vi "2.vi"() -> ()   [LabVIEW 2019]
uses:
  <vilib>/imath/engines/lvmath/Plug In/_Char/NIMS_CH_character datatype.ctl
  <vilib>/imath/engines/lvmath2/RunTimeEngine/RangeToken/NIMS_Range.vi
  <instcachedir>/0/NIMS_Range_FADF6ADDA3E145BB934C8BD4C7DAAB97.lvgen/NIMS_Range_FADF6ADDA3E145BB934C8BD4C7DAAB97_000.vi
  <vilib>/imathl/engines/lvmath/Functions/Error Handling/Create Error.vi
  <vilib>/imath/engines/lvmath/Plug In/_Char/NIMS_CH_Character RV to String.vi
  <vilib>/imath/engines/lvmath2/RunTimeEngine/BuiltInFunctions/random/NIMS_random.vi
  <vilib>/imath/engines/lvmath2/RunTimeEngine/IndexRead/NIMS M(S).vi
  <instcachedir>/0/NIMS M(S)_B826C018497E4940AE96BD27B540B6FB.lvgen/NIMS M(S)_B826C018497E4940AE96BD27B540B6FB_000.vi
  <vilib>/imath/engines/lvmath2/RunTimeEngine/ArithmeticOperatorToken/NIMS_ArithmeticOperator_plus.vi
  <instcachedir>/0/NIMS_ArithmeticOperator_plus_5C9385B0197D46E2B844C41E02F9EC39.lvgen/NIMS_ArithmeticOperator_plus_5C9385B0197D46E2B844C41E02F9EC39_004.vi
  <vilib>/imath/engines/lvmath2/RunTimeEngine/ErrorHandling/NIMS_Create Error From Enums.vi
  <vilib>/imath/engines/lvmath2/RunTimeEngine/BuiltInFunctions/randnormal/NIMS_randnormal(1,I32).vi
  <vilib>/imath/engines/lvmath2/RunTimeEngine/ErrorHandling/NIMS_Error From Error Code.vi
  <vilib>/imath/engines/lvmath/Functions/Error Handling/MergeErrorsWrapper.vi
  <vilib>/imath/engines/lvmath2/RunTimeEngine/BuiltInFunctions/crosscorr/NIMS_crosscorr(GM,Str).vi
  <instcachedir>/0/NIMS_crosscorr(GM,Str)_7E3A3CE9917B451394D0C3CD4C3D6955.lvgen/NIMS_crosscorr(GM,Str)_7E3A3CE9917B451394D0C3CD4C3D6955_000.vi
  <vilib>/imath/engines/lvmath2/RunTimeEngine/BuiltInFunctions/fft/NIMS_fft(GM).vi
  <instcachedir>/0/NIMS_fft(GM)_17D9014FFEBE444196AC5CE36A7D9342.lvgen/NIMS_fft(GM)_17D9014FFEBE444196AC5CE36A7D9342_000.vi
  <vilib>/imath/engines/lvmath2/RunTimeEngine/BuiltInFunctions/abs/NIMS_abs(signed).vi
  <instcachedir>/0/NIMS_abs(signed)_C4FCB8E6058B49B797C7C8D53CA5F6EC.lvgen/NIMS_abs(signed)_C4FCB8E6058B49B797C7C8D53CA5F6EC_003.vi
  <vilib>/imath/engines/lvmath2/RunTimeSupport/NIMS_Error if Not Equal.vi
  <instcachedir>/0/NIMS_Error if Not Equal_D50A0F08CBFC40E0B64682CCD852CBC7.lvgen/NIMS_Error if Not Equal_D50A0F08CBFC40E0B64682CCD852CBC7_001.vi
  <vilib>/imath/engines/lvmath2/RunTimeEngine/IndexRead/NIMS M(V).vi
  <instcachedir>/0/NIMS M(V)_948FAC22C1C943948B75DA6190348614.lvgen/NIMS M(V)_948FAC22C1C943948B75DA6190348614_004.vi
  <instcachedir>/0/NIMS M(V)_948FAC22C1C943948B75DA6190348614.lvgen/NIMS M(V)_948FAC22C1C943948B75DA6190348614_005.vi
  <vilib>/imath/engines/lvmath2/RunTimeEngine/BuiltInFunctions/plot/NIMS_plot(RM, RM, Str).vi
  <vilib>/imath/engines/lvmath2/RunTimeEngine/BuiltInFunctions/grid/NIMS_grid(Enums).vi
  <vilib>/imath/engines/lvmath2/RunTimeEngine/BuiltInFunctions/psd/NIMS_psd().vi
  <instcachedir>/0/NIMS_psd()_DD28FF9C416C4982A5CB7EF3090E8523.lvgen/NIMS_psd()_DD28FF9C416C4982A5CB7EF3090E8523_000.vi
  <vilib>/imath/engines/lvmath2/RunTimeEngine/BuiltInFunctions/psd_welch/NIMS_psd_welch().vi
  <instcachedir>/0/NIMS_psd_welch()_DC42BB47114F48A099E10F6AAAA25512.lvgen/NIMS_psd_welch()_DC42BB47114F48A099E10F6AAAA25512_000.vi
  <vilib>/imath/engines/lvmath2/RunTimeEngine/NodeEndStatement/NIMS_NodeEndStatement_Get Vector.vi
  <instcachedir>/0/NIMS_NodeEndStatement_Get Vector_92F29E6578CC4FEABDAC0B727A70E862.lvgen/NIMS_NodeEndStatement_Get Vector_92F29E6578CC4FEABDAC0B727A70E862_003.vi
  <vilib>/imath/engines/lvmath2/RunTimeEngine/NodeEndStatement/NIMS_NodeEndStatement_Output.vi
  <instcachedir>/0/NIMS_NodeEndStatement_Output_53EC0D466D134D7ABD903AC30B43404B.lvgen/NIMS_NodeEndStatement_Output_53EC0D466D134D7ABD903AC30B43404B_005.vi
  <vilib>/imath/engines/lvmath2/RunTimeEngine/ErrorHandling/NIMS_Finalize Error.vi
panel:
  out "psd函数估计功率谱":cluster{"f":dbl[], "logsx2":dbl[]}(graph)
  out "Welch函数估计功率谱":cluster{"f":dbl[], "logsx3":dbl[]}(graph)
  out "自相关函数法估计功率谱":cluster{"f1":dbl[], "logsx1":dbl[]}(graph)
  out "随机信号时域波形":dbl[](graph)
  in  "A2":dbl=5.0
  in  "A1":dbl=2.0
  in  "f2":dbl=100.0
  in  "f1":dbl=30.0
  in  "fs":dbl=1000.0
  in  "N":dbl=1024.0
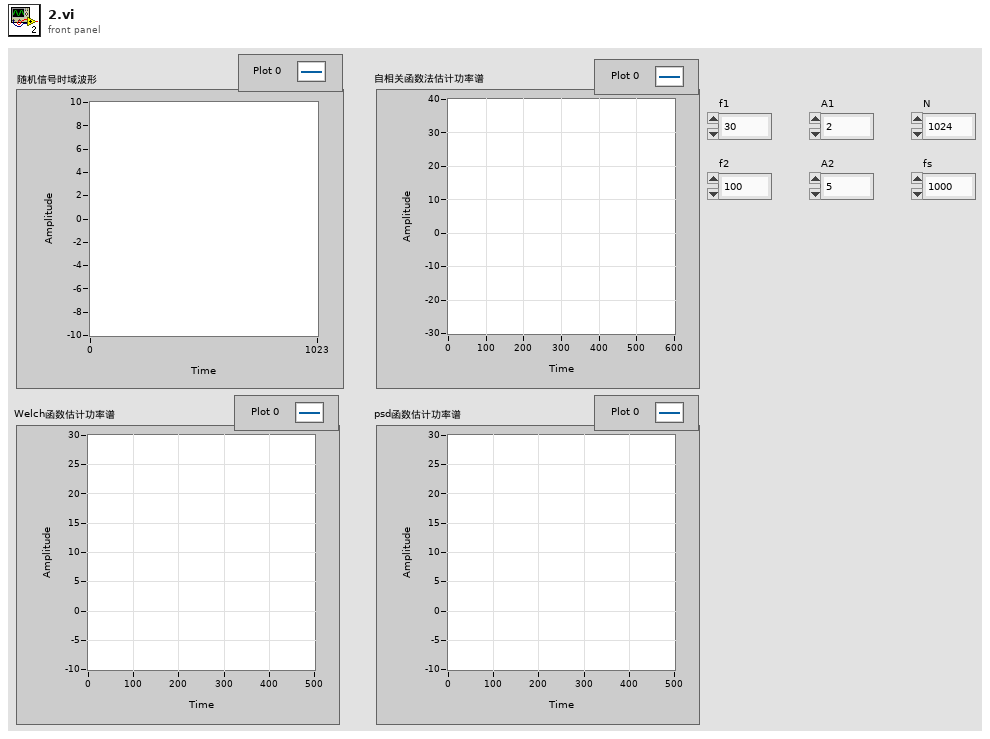
[diagram p1: front panel]
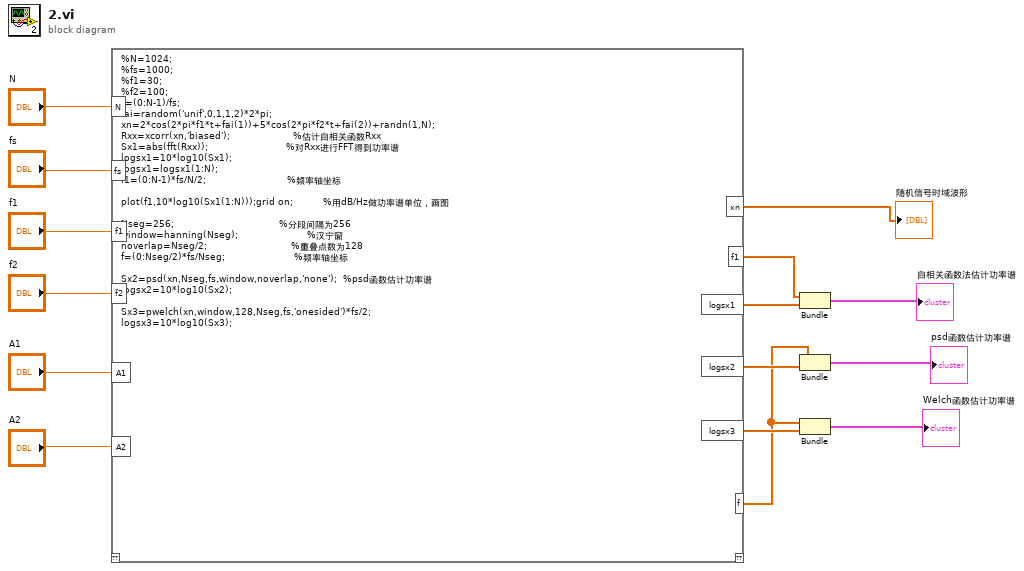
[diagram p0: block diagram]
diagram:
  n1 = mathscript code="%N=1024;\n%fs=1000;\n%f1=30;\n%f2=100;\nt=(0:N-1)/fs;\nfai=random('unif',0,1,1,2)*2*pi;\nxn=2*cos(2*pi*f1*t+fai(1))+5*cos(2*pi*f2*t+fai(2))+randn(1,N);\nRxx=xcorr(xn,'biased');                     %估计自相关函数Rxx\nSx1=abs(fft(Rxx));                          %对Rxx进行FFT得到功率谱\nlogsx1=10*log10(Sx1);\nlogsx1=logsx1(1:N);\nf1=(0:N-1)*fs/N/2;                           %频率轴坐标\n\nplot(f1,10*log10(Sx1(1:N)));grid on;          %用dB/Hz做功率谱单位，画图\n\nNseg=256;                                   %分段间隔为256\nwindow=hanning(Nseg);                       %汉宁窗\nnoverlap=Nseg/2;                            %重叠点数为128\nf=(0:Nseg/2)*fs/Nseg;                       %频率轴坐标\n\nSx2=psd(xn,Nseg,fs,window,noverlap,'none');  %psd函数估计功率谱\nlogsx2=10*log10(Sx2);\n\nSx3=pwelch(xn,window,128,Nseg,fs,'onesided')*fs/2;\nlogsx3=10*log10(Sx3);"("N"="N", "fs"="fs", "f1"="f1", "f2"="f2", "A1"="A1", "A2"="A2") -> ("xn"=→"随机信号时域波形":dbl[], "logsx1"=w9:dbl[], "logsx2"=w8:dbl[], "logsx3"=w7:dbl[], "f"=w6:dbl[], "f1"=w5:dbl[])  [unwired: 1 in, 1 out]
  n2 = Bundle("f1"=w5, "logsx1"=w9) -> (→"自相关函数法估计功率谱":cluster{"f1":dbl[], "logsx1":dbl[]})  [unwired: 1 in]
  n3 = Bundle("f"=w6, "logsx2"=w8) -> (→"psd函数估计功率谱":cluster{"f":dbl[], "logsx2":dbl[]})  [unwired: 1 in]
  n4 = Bundle("f"=w6, "logsx3"=w7) -> (→"Welch函数估计功率谱":cluster{"f":dbl[], "logsx3":dbl[]})  [unwired: 1 in]
